vi "LoadDefaults.vi"(8 "error in (no error)":errorcluster, 11 "ThorlabsLabJack in":refnum<class "ThorlabsLabJack.lvclass">) -> (0 "error out":errorcluster, 3 "ThorlabsLabJack out":refnum<class "ThorlabsLabJack.lvclass">)   [LabVIEW 2018, in "ThorlabsLabJack.lvlib" / "ThorlabsLabJack.lvclass"]
uses:
  ThorlabsLabJack.lvclass
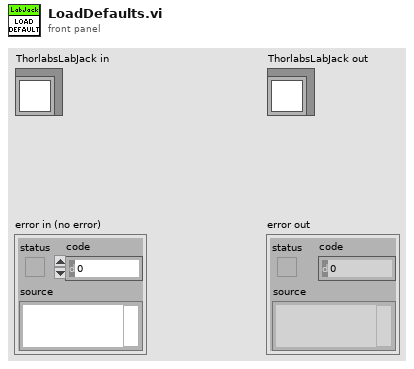
[diagram p1: front panel]
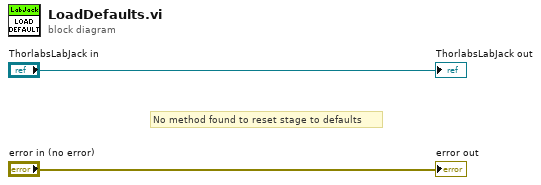
[diagram p0: block diagram]
diagram:
  # "No method found to reset stage to defaults"
  "error out" <- "error in (no error)"
  "ThorlabsLabJack out" <- "ThorlabsLabJack in"
